vi "build.proc.parse.vi"(8 "error":errorcluster, 11 "Array in":variant[](array[variant])) -> (0 "error out":errorcluster, 2 "Flow Steps":T1[](array[typedef]), 3 "Proc Head":T3)   [LabVIEW 2024]
uses:
  controls/UiProcHeader.ctl
  controls/UiStepBuilder.ctl
  controls/type.step-builder.ctl
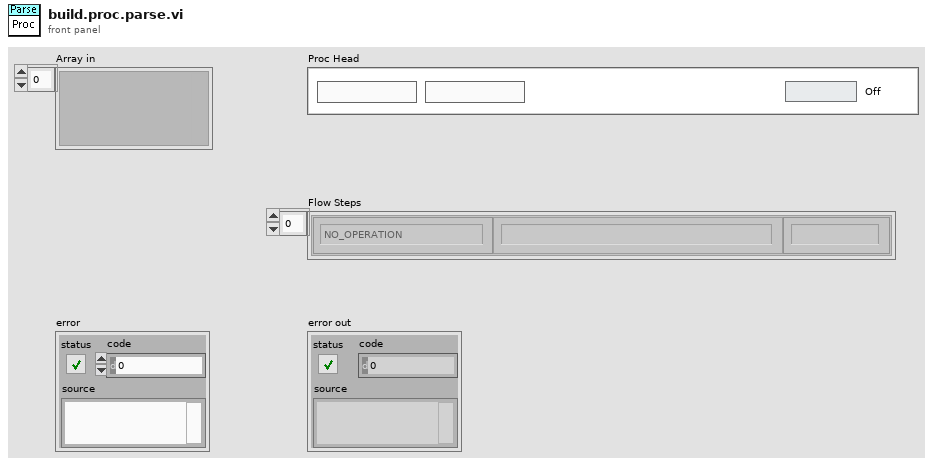
[diagram p1: front panel]
types:
  T1 = typedef "UiStepBuilder.ctl" = cluster{"Step Function":T2, "ParamString":string, "Step Label":string}
  T2 = typedef "type.step-builder.ctl" = enum16{"NO_OPERATION", "DELAY-JUMP", "DELAY", "JUMP", "COMPLETE", "SCHEDULER", "IRR-CHECK", "UNIT-CHECK", "UNIT-SAMPLE", "UNIT-DOSE", "LOG-REPORT", "LOG-MESSAGE", "IO-READ", "IO-READ-MANY", "IO-WRITE", "IO-COMPARE-OUT", "IO-COMPARE-IN", "PROC-START", "PROC-STOP", "PROC-LOAD", "PROC-IS-COMPLETED", "RECORD-MOVE", "GET-RH", "GET-UV", "GET-WD", "GET-WS", "OCS-CHECK", "OCS-RECORD"}
  T3 = typedef "UiProcHeader.ctl" = cluster{"Procedure Name":string, "Running":bool, "tags":string}
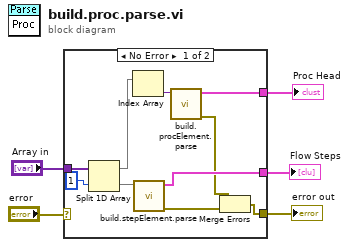
[diagram p0: block diagram]
diagram:
  n1 = case shown="No Error" "error" {
    selector: "error" -> [_ w16]
    tunnel: "Array in" -> [w11 _]
    tunnel: [w10 _] -> w4
    tunnel: [w9 _] -> w3
    tunnel: [w7 w16] -> w2
    frame No Error {
      n2 = Split 1D Array(array=w11, index=1) -> (first subarray=w12:variant[], second subarray=w15:variant[])
      n3 = Index Array(array=w12) -> (element=w14:variant)  [unwired: 1 in]
      n4 = call "build.stepElement.parse.vi"("steps in"=w15) -> ("error out"=w8:errorcluster, "Flow Elements"=w9:T1[])  [unwired: 9 in]
      n5 = call "build.procElement.parse.vi"("procElement in"=w14) -> ("error out"=w6:errorcluster, "UiBuildProcHead"=w10:T3)  [unwired: 9 in]
      n6 = Merge Errors(w6, w8) -> (w7:errorcluster)
    }
    frame Error {
    }
  }
  "Proc Head" <- w4
  "Flow Steps" <- w3
  "error out" <- w2
